vi "Weather_Settings_to_Queue.vi"(0 "GPS time difference":i32, 1 "Current PC time":timestamp) -> ()   [LabVIEW 2013]
uses:
  Globals/Ini_Files.vi
  <vilib>/Utility/config.llb/Read Key (I32).vi
  <vilib>/Utility/config.llb/Read Key (String).vi
  <vilib>/Utility/config.llb/Read Key (Boolean).vi
  <vilib>/Utility/config.llb/Read Key (Double).vi
  Globals/Weather_Queues.vi
  <vilib>/Utility/config.llb/NI_LVConfig.lvlib
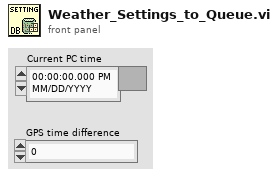
[diagram p1: front panel]
types:
  T1 = cluster{"Path Run Status file":path, "Path Default Settings file":path, "Path User Settings file":path}
  T2 = typedef "NI_LVConfig.lvlib/Config Data RefNum.ctl" = refnum<k1>
  T3 = cluster{"Weather data (5s)":refnum<queue>, "Database queue":refnum<queue>, "Message queue":refnum<queue>, "Settings queue":refnum<queue>, "60 mins data queue":refnum<queue>, "48 hrs data queue":refnum<queue>}
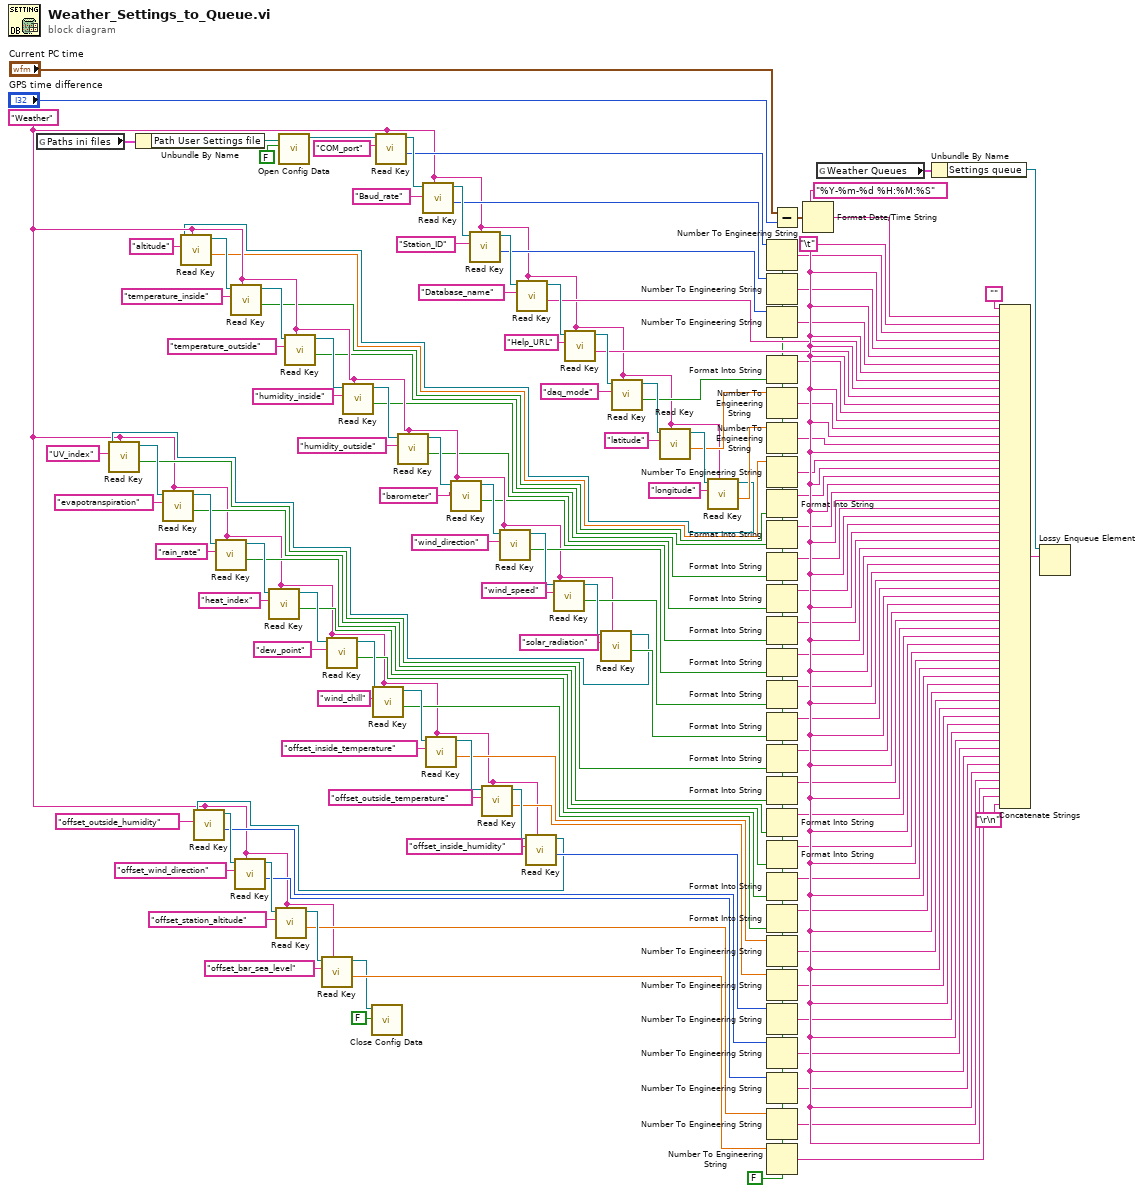
[diagram p0: block diagram]
diagram:
  w1 = FALSE ("use system decimal point (T)")
  w136 = "\t"
  w13 = "Weather" ("section")
  n1 = global read "Ini_Files.vi" "Paths ini files"() -> (w21:T1)
  n2 = Unbundle By Name(w21) -> ("Path User Settings file"=w27:path)
  n3 = call <vilib>:"Open Config Data.vi"("create file if necessary (T)"=FALSE, "configuration file path"=w27) -> ("refnum"=w126:T2)  [unwired: 7 in, 2 out]
  n4 = call-poly <vilib>:"Read Key.vi"("section"=w13, "key"="COM_port", "refnum"=w126) -> ("value"=w86:i32, "refnum out"=w125:T2)  [unwired: 5 in, 2 out]
  n5 = call-poly <vilib>:"Read Key.vi"("section"=w13, "key"="Baud_rate", "refnum"=w125) -> ("value"=w84:i32, "refnum out"=w99:T2)  [unwired: 5 in, 2 out]
  n6 = call-poly <vilib>:"Read Key.vi"("section"=w13, "key"="Station_ID", "refnum"=w99) -> ("value"=w83:i32, "refnum out"=w98:T2)  [unwired: 5 in, 2 out]
  n7 = call-poly <vilib>:"Read Key.vi"("section"=w13, "key"="Database_name" ("Key name"), "refnum"=w98) -> ("value"=w82:string, "refnum out"=w97:T2)  [unwired: 5 in, 2 out]
  n8 = call-poly <vilib>:"Read Key.vi"("section"=w13, "key"="Help_URL" ("Key name"), "refnum"=w97) -> ("value"=w81:string, "refnum out"=w96:T2)  [unwired: 5 in, 2 out]
  n9 = call-poly <vilib>:"Read Key.vi"("section"=w13, "key"="daq_mode", "refnum"=w96) -> ("value"=w79:bool, "refnum out"=w95:T2)  [unwired: 5 in, 2 out]
  n10 = call-poly <vilib>:"Read Key.vi"("section"=w13, "key"="latitude", "refnum"=w95) -> ("value"=w78:dbl, "refnum out"=w94:T2)  [unwired: 5 in, 2 out]
  n11 = call-poly <vilib>:"Read Key.vi"("section"=w13, "key"="longitude", "refnum"=w94) -> ("value"=w77:dbl, "refnum out"=w4:T2)  [unwired: 5 in, 2 out]
  n12 = call-poly <vilib>:"Read Key.vi"("section"=w13, "key"="altitude", "refnum"=w4) -> ("value"=w10:dbl, "refnum out"=w12:T2)  [unwired: 5 in, 2 out]
  n13 = call-poly <vilib>:"Read Key.vi"("section"=w13, "key"="temperature_inside", "refnum"=w12) -> ("value"=w5:bool, "refnum out"=w93:T2)  [unwired: 5 in, 2 out]
  n14 = call-poly <vilib>:"Read Key.vi"("section"=w13, "key"="temperature_outside", "refnum"=w93) -> ("value"=w6:bool, "refnum out"=w92:T2)  [unwired: 5 in, 2 out]
  n15 = call-poly <vilib>:"Read Key.vi"("section"=w13, "key"="humidity_inside", "refnum"=w92) -> ("value"=w7:bool, "refnum out"=w91:T2)  [unwired: 5 in, 2 out]
  n16 = call-poly <vilib>:"Read Key.vi"("section"=w13, "key"="humidity_outside", "refnum"=w91) -> ("value"=w8:bool, "refnum out"=w90:T2)  [unwired: 5 in, 2 out]
  n17 = call-poly <vilib>:"Read Key.vi"("section"=w13, "key"="barometer", "refnum"=w90) -> ("value"=w9:bool, "refnum out"=w89:T2)  [unwired: 5 in, 2 out]
  n18 = call-poly <vilib>:"Read Key.vi"("section"=w13, "key"="wind_direction", "refnum"=w89) -> ("value"=w70:bool, "refnum out"=w88:T2)  [unwired: 5 in, 2 out]
  n19 = call-poly <vilib>:"Read Key.vi"("section"=w13, "key"="wind_speed", "refnum"=w88) -> ("value"=w68:bool, "refnum out"=w87:T2)  [unwired: 5 in, 2 out]
  n20 = call-poly <vilib>:"Read Key.vi"("section"=w13, "key"="solar_radiation", "refnum"=w87) -> ("value"=w69:bool, "refnum out"=w23:T2)  [unwired: 5 in, 2 out]
  n21 = call-poly <vilib>:"Read Key.vi"("section"=w13, "key"="UV_index", "refnum"=w23) -> ("value"=w24:bool, "refnum out"=w60:T2)  [unwired: 5 in, 2 out]
  n22 = call-poly <vilib>:"Read Key.vi"("section"=w13, "key"="evapotranspiration", "refnum"=w60) -> ("value"=w25:bool, "refnum out"=w59:T2)  [unwired: 5 in, 2 out]
  n23 = call-poly <vilib>:"Read Key.vi"("section"=w13, "key"="rain_rate", "refnum"=w59) -> ("value"=w55:bool, "refnum out"=w58:T2)  [unwired: 5 in, 2 out]
  n24 = call-poly <vilib>:"Read Key.vi"("section"=w13, "key"="heat_index", "refnum"=w58) -> ("value"=w51:bool, "refnum out"=w57:T2)  [unwired: 5 in, 2 out]
  n25 = call-poly <vilib>:"Read Key.vi"("section"=w13, "key"="dew_point", "refnum"=w57) -> ("value"=w50:bool, "refnum out"=w56:T2)  [unwired: 5 in, 2 out]
  n26 = call-poly <vilib>:"Read Key.vi"("section"=w13, "key"="wind_chill", "refnum"=w56) -> ("value"=w49:bool, "refnum out"=w54:T2)  [unwired: 5 in, 2 out]
  n27 = call-poly <vilib>:"Read Key.vi"("section"=w13, "key"="offset_inside_temperature", "refnum"=w54) -> ("value"=w48:dbl, "refnum out"=w53:T2)  [unwired: 5 in, 2 out]
  n28 = call-poly <vilib>:"Read Key.vi"("section"=w13, "key"="offset_outside_temperature", "refnum"=w53) -> ("value"=w47:dbl, "refnum out"=w52:T2)  [unwired: 5 in, 2 out]
  n29 = call-poly <vilib>:"Read Key.vi"("section"=w13, "key"="offset_inside_humidity", "refnum"=w52) -> ("value"=w46:i32, "refnum out"=w22:T2)  [unwired: 5 in, 2 out]
  n30 = call-poly <vilib>:"Read Key.vi"("section"=w13, "key"="offset_outside_humidity", "refnum"=w22) -> ("value"=w39:i32, "refnum out"=w42:T2)  [unwired: 5 in, 2 out]
  n31 = call-poly <vilib>:"Read Key.vi"("section"=w13, "key"="offset_wind_direction", "refnum"=w42) -> ("value"=w38:i32, "refnum out"=w41:T2)  [unwired: 5 in, 2 out]
  n32 = call-poly <vilib>:"Read Key.vi"("section"=w13, "key"="offset_station_altitude", "refnum"=w41) -> ("value"=w37:dbl, "refnum out"=w40:T2)  [unwired: 5 in, 2 out]
  n33 = call-poly <vilib>:"Read Key.vi"("section"=w13, "key"="offset_bar_sea_level", "refnum"=w40) -> ("value"=w36:dbl, "refnum out"=w2:T2)  [unwired: 5 in, 2 out]
  n34 = call <vilib>:"Close Config Data.vi"("write file if changed (T)"=FALSE, "refnum"=w2) -> ()  [unwired: 8 in, 2 out]
  n35 = Number To Engineering String(1:w1, 4:w86) -> (0:w85:string)  [unwired: 2 out]
  n36 = Number To Engineering String(1:w1, 4:w84) -> (0:w101:string)  [unwired: 2 out]
  n37 = Number To Engineering String(1:w1, 4:w83) -> (0:w100:string)  [unwired: 2 out]
  n38 = Format Into String(w79) -> (resulting string=w80:string)  [unwired: 3 in, 1 out]
  n39 = Number To Engineering String(1:w1, 4:w78) -> (0:w103:string)  [unwired: 2 out]
  n40 = Number To Engineering String(1:w1, 4:w77) -> (0:w102:string)  [unwired: 2 out]
  n41 = Number To Engineering String(1:w1, 4:w10) -> (0:w11:string)  [unwired: 2 out]
  n42 = Format Into String(w5) -> (resulting string=w3:string)  [unwired: 3 in, 1 out]
  n43 = Format Into String(w6) -> (resulting string=w76:string)  [unwired: 3 in, 1 out]
  n44 = Format Into String(w7) -> (resulting string=w71:string)  [unwired: 3 in, 1 out]
  n45 = Format Into String(w8) -> (resulting string=w72:string)  [unwired: 3 in, 1 out]
  n46 = Format Into String(w9) -> (resulting string=w73:string)  [unwired: 3 in, 1 out]
  n47 = Format Into String(w70) -> (resulting string=w74:string)  [unwired: 3 in, 1 out]
  n48 = Format Into String(w68) -> (resulting string=w75:string)  [unwired: 3 in, 1 out]
  n49 = Format Into String(w69) -> (resulting string=w67:string)  [unwired: 3 in, 1 out]
  n50 = Format Into String(w24) -> (resulting string=w66:string)  [unwired: 3 in, 1 out]
  n51 = Format Into String(w25) -> (resulting string=w65:string)  [unwired: 3 in, 1 out]
  n52 = Format Into String(w55) -> (resulting string=w64:string)  [unwired: 3 in, 1 out]
  n53 = Format Into String(w51) -> (resulting string=w63:string)  [unwired: 3 in, 1 out]
  n54 = Format Into String(w50) -> (resulting string=w62:string)  [unwired: 3 in, 1 out]
  n55 = Format Into String(w49) -> (resulting string=w61:string)  [unwired: 3 in, 1 out]
  n56 = Number To Engineering String(1:w1, 4:w48) -> (0:w45:string)  [unwired: 2 out]
  n57 = Number To Engineering String(1:w1, 4:w47) -> (0:w44:string)  [unwired: 2 out]
  n58 = Number To Engineering String(1:w1, 4:w46) -> (0:w43:string)  [unwired: 2 out]
  n59 = Number To Engineering String(1:w1, 4:w39) -> (0:w35:string)  [unwired: 2 out]
  n60 = Number To Engineering String(1:w1, 4:w38) -> (0:w34:string)  [unwired: 2 out]
  n61 = Number To Engineering String(1:w1, 4:w37) -> (0:w33:string)  [unwired: 2 out]
  n62 = Number To Engineering String(1:w1, 4:w36) -> (0:w32:string)  [unwired: 2 out]
  n63 = Subtract(x="Current PC time", y="GPS time difference") -> (x-y=w17:timestamp)
  n64 = Format Date/Time String(time format string (%c)="%Y-%m-%d %H:%M:%S", seconds (now)=w17) -> (date/time string=w18:string)  [unwired: 1 out]
  n65 = global read "Weather_Queues.vi" "Weather Queues"() -> (w26:T3)
  n66 = Unbundle By Name(w26) -> ("Settings queue"=w28:refnum<queue>)
  n67 = Concatenate Strings("", w18, w136, w85, w136, w101, w136, w100, w136, w82, w136, w81, w136, w80, w136, w103, w136, w102, w136, w11, w136, w3, w136, w76, w136, w71, w136, w72, w136, w73, w136, w74, w136, w75, w136, w67, w136, w66, w136, w65, w136, w64, w136, w63, w136, w62, w136, w61, w136, w45, w136, w44, w136, w43, w136, w35, w136, w34, w136, w33, w136, w32, "\r\n") -> (w31:string)
  n68 = Lossy Enqueue Element(queue=w28, element=w31) -> ()  [unwired: 1 in, 4 out]
